vi "GetTeamsList.vi"() -> (3 "Array":cluster{string, "value":string}[](array[cluster]))   [LabVIEW 2017]
uses:
  <vilib>/Utility/config.llb/Read Key (String).vi
  <vilib>/Utility/config.llb/NI_LVConfig.lvlib
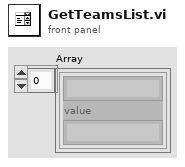
[diagram p1: front panel]
types:
  T1 = typedef "NI_LVConfig.lvlib/Config Data RefNum.ctl" = refnum<k1>
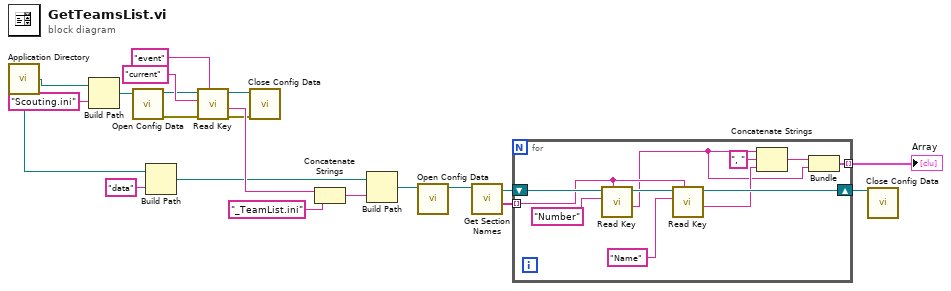
[diagram p0: block diagram]
diagram:
  n1 = call <vilib>:"Application Directory.vi"() -> ("Application Directory"=w20:path)
  n2 = Build Path(base path=w20, name or relative path="Scouting.ini") -> (appended path=w7:path)
  n3 = call <vilib>:"Open Config Data.vi"("configuration file path"=w7) -> ("error out"=w1:errorcluster, "refnum"=w2:T1)  [unwired: 8 in, 1 out]
  n4 = Build Path(base path=w20, name or relative path="data") -> (appended path=w9:path)
  n5 = call-poly <vilib>:"Read Key.vi"("section"="event" ("key"), "error in (no error)"=w1, "key"="current" ("section"), "refnum"=w2) -> ("error out"=w3:errorcluster, "value"=w11:string, "refnum out"=w4:T1)  [unwired: 4 in, 1 out]
  n6 = call <vilib>:"Close Config Data.vi"("error in (no error)"=w3, "refnum"=w4) -> ()  [unwired: 8 in, 2 out]
  n7 = Concatenate Strings(w11, "_TeamList.ini" ("string")) -> (w10:string)
  n8 = Build Path(base path=w9, name or relative path=w10) -> (appended path=w14:path)
  n9 = call <vilib>:"Open Config Data.vi"("configuration file path"=w14) -> ("refnum"=w15:T1)  [unwired: 8 in, 2 out]
  n10 = call <vilib>:"Get Section Names.vi"("refnum"=w15) -> ("section names"=w16:string[], "refnum out"=w17:T1)  [unwired: 8 in, 1 out]
  n11 = for {
    tunnel: w16 -> [w28] mode=indexing
    shift-right: [w26] -> w19
    shift-left: w17 -> [w31]
    tunnel: [w25] -> w18 mode=indexing
    n12 = call-poly <vilib>:"Read Key.vi"("section"=w28, "key"="Number", "refnum"=w31) -> ("value"=w21:string, "refnum out"=w29:T1)  [unwired: 5 in, 2 out]
    n13 = call-poly <vilib>:"Read Key.vi"("section"=w28, "key"="Name", "refnum"=w29) -> ("value"=w24:string, "refnum out"=w26:T1)  [unwired: 5 in, 2 out]
    n14 = Concatenate Strings(w21, ", " ("string"), w24) -> (w22:string)
    n15 = Bundle(w22, "value"=w21) -> (w25:cluster{string, "value":string})  [unwired: 1 in]
  }
  "Array" <- w18
  n16 = call <vilib>:"Close Config Data.vi"("refnum"=w19) -> ()  [unwired: 9 in, 2 out]
